vi "Load.vi"(8 "error in (no error)":errorcluster, 10 "Vi Path":path=path "C:/Users/namratha.balakrishna/Documents/LabVIEW Data/MDI/source code/Labview MDI/Example/Waveform.vi", 11 "LV MDI in":refnum<class "LV MDI.lvclass">) -> (0 "error out":errorcluster, 3 "LV MDI out":refnum<class "LV MDI.lvclass">)   [LabVIEW 2016, in "LV MDI.lvclass"]
uses:
  LV MDI.lvclass
  LV MDI.lvclass/LV MDI.ctl
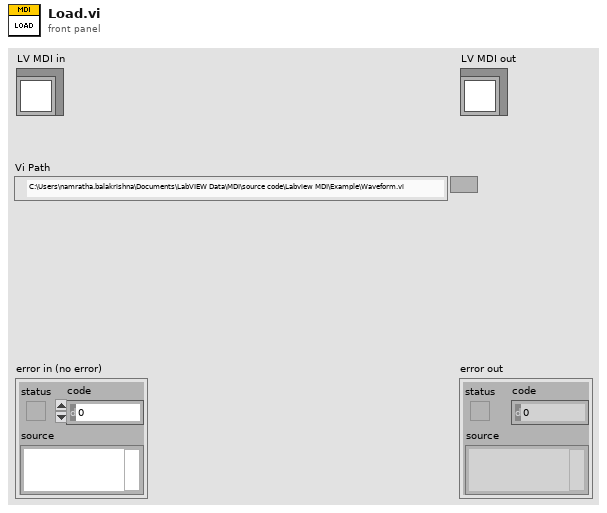
[diagram p1: front panel]
types:
  T1 = typedef "LV MDI.lvclass/Window Data.ctl" = cluster{"Child hWnd":u32, "UID":string, "vi reference":refnum<vi>, "Name":string}
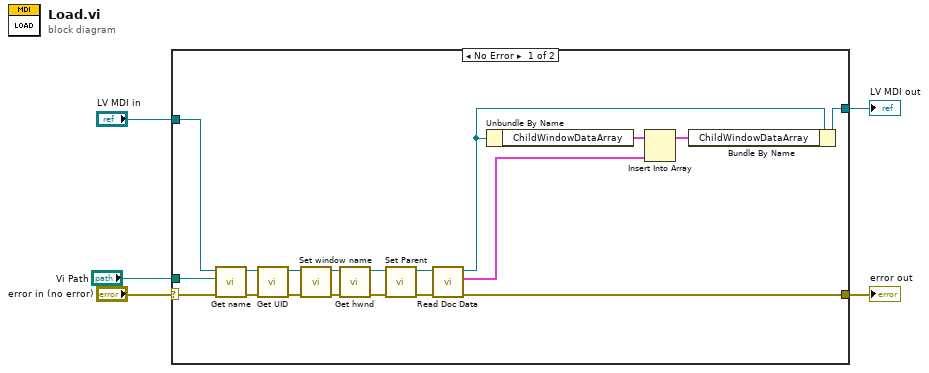
[diagram p0: block diagram]
diagram:
  n1 = case shown="No Error" "error in (no error)" {
    selector: "error in (no error)" -> [w23 w26]
    tunnel: [w11 w26] -> w4
    tunnel: [w6 w25] -> w2
    tunnel: "LV MDI in" -> [w21 w25]
    tunnel: "Vi Path" -> [w22 _]
    frame No Error {
      n2 = call "Get name.vi"("Error in"=w23, "Vi Path"=w22, "LV MDI in"=w21) -> ("Error Out"=w24:errorcluster, "LV MDI out"=w20:refnum<class "LV MDI.lvclass">)  [unwired: 7 in]
      n3 = call "Get UID.vi"("error in (no error)"=w24, "LV MDI in"=w20) -> ("error out"=w18:errorcluster, "LV MDI out"=w19:refnum<class "LV MDI.lvclass">)  [unwired: 8 in]
      n4 = call "Set window name.vi"("error in (no error)"=w18, "LV MDI in"=w19) -> ("error out"=w17:errorcluster, "LV MDI out"=w16:refnum<class "LV MDI.lvclass">)  [unwired: 8 in]
      n5 = call "Get hwnd.vi"("Error in"=w17, "LV MDI.lvclass"=w16) -> ("Error Out"=w14:errorcluster, "LV MDI.lvclass  2"=w15:refnum<class "LV MDI.lvclass">)  [unwired: 8 in]
      n6 = call "Set Parent.vi"("error in (no error)"=w14, "LV MDI in"=w15) -> ("error out"=w12:errorcluster, "LV MDI out"=w13:refnum<class "LV MDI.lvclass">)  [unwired: 8 in]
      n7 = call-dynamic "Read Doc Data.vi"("error in (no error)"=w12, "LV MDI.lvclass"=w13) -> ("error out"=w11:errorcluster, "Child Window Data"=w9:T1, "LV MDI.lvclass"=w7:refnum<class "LV MDI.lvclass">)  [unwired: 7 in]
      n8 = Unbundle By Name(w7) -> ("ChildWindowDataArray"=w10:T1[])
      n9 = Insert Into Array(array=w10, new element=w9) -> (w8:T1[])  [unwired: 1 in]
      n10 = Bundle By Name(cluster=w7, "ChildWindowDataArray"=w8) -> (w6:refnum<class "LV MDI.lvclass">)
    }
    frame Error {
    }
  }
  "error out" <- w4
  "LV MDI out" <- w2
